vi "poke.vi"(6 "timeout (25000ms)":i32=25000, 8 "error in (no error)":errorcluster, 9 "data":i32, 10 "parameter name":string, 11 "daemon reference in":refnum<k5>) -> (0 "error out":errorcluster, 2 "response":string, 3 "daemon reference out":refnum<k5>, 5 "command out":string="random")   [LabVIEW 2017]
doc: "<b>Command: </b>\"poke\"\n\n<b>Description: </b>This command pokes a variable stored in memory on the target in an attempt to overwrite the value stored.\n\n<b>Parameters: </b> \n\n 1. Name of variable to poke\n 2. Numeric representing value to be stored\n\n<b>Note: </b>This command will only work on DEV builds of the target and as long as the relevant firmware json file has been loaded using \"load_firmware_json\" command.\n____________________________________________\nDIPC 692 Daemon API 10.0.0.1\nSam Tee - Dyson Technology Ltd\nCopyright (c) 2024, Dyson Technology Ltd"
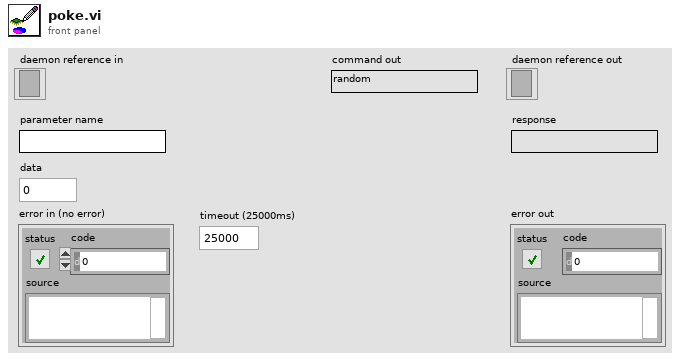
[diagram p1: front panel]
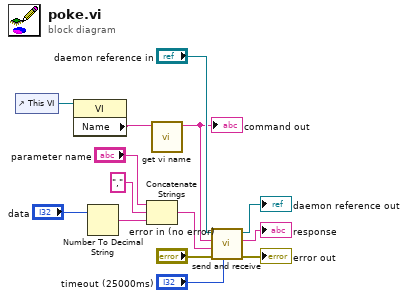
[diagram p0: block diagram]
diagram:
  n1 = control-ref of="This VI"() -> (w9:refnum<vi>)
  n2 = property class="VI"(reference=w9) -> ("Name"=w7:string)  [unwired: 1 in, 2 out]
  n3 = Number To Decimal String(number="data") -> (decimal integer string=w2:string)  [unwired: 1 in]
  n4 = Concatenate Strings("parameter name", "," ("string"), w2) -> (w5:string)
  n5 = call "get vi name.vi"("library.lvlib:name.vi"=w7) -> ("vi name"=w6:string)  [unwired: 10 in]
  "command out" <- w6
  n6 = call "send and receive.vi"("timeout (25000ms)"="timeout (25000ms)", "error in (no error)"="error in (no error)", "data"=w5, "command"=w6, "daemon reference in"="daemon reference in") -> ("error out"=→"error out":errorcluster, "response"=→"response":string, "daemon reference out"=→"daemon reference out":refnum<k5>)  [unwired: 4 in]
